vi "SampleGetIDMultiple.vi"() -> ()   [LabVIEW 2016]
panel:
  out "Device number":i32
  out "Identification List":string[](array[string])
  out "DeviceKey List Out":string[](array[string])
  out "error out":errorcluster
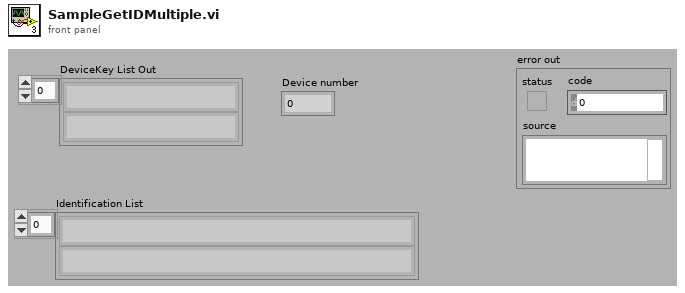
[diagram p1: front panel]
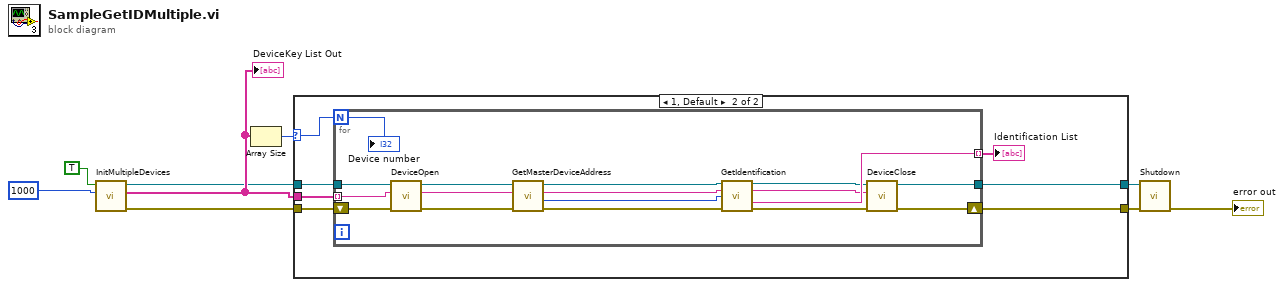
[diagram p0: block diagram]
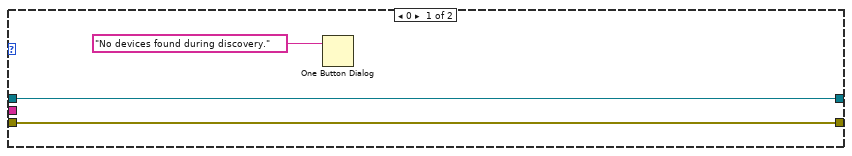
[diagram p2: hidden frame]
diagram:
  n1 = call "InitMultipleDevices.vi"("msecDelayForDiscovery"=1000, "logging"=TRUE) -> ("error out"=w1:errorcluster, "DeviceKey List Out"=w5:string[], "CmdLib Out"=w2:refnum<k24>)  [unwired: 3 in]
  "DeviceKey List Out" <- w5
  n2 = Array Size(array=w5) -> (size(s)=w6:i32)
  n3 = case shown="1, Default" w6 {
    selector: w6 -> [_ w19]
    tunnel: w5 -> [_ w18]
    tunnel: w2 -> [w11 w17]
    tunnel: w1 -> [w12 w16]
    tunnel: [w12 w15] -> w4
    tunnel: [w11 w14] -> w3
    frame 0 {
      n4 = One Button Dialog(message="No devices found during discovery.") -> ()  [unwired: 1 in, 1 out]
    }
    frame 1, Default {
      n5 = for {
        N: w19 -> [w20]
        tunnel: w18 -> [w32] mode=indexing
        tunnel: [w36] -> w13 mode=indexing
        tunnel: w17 -> [w35]
        tunnel: [w34] -> w14
        shift-right: [w30] -> w15
        shift-left: w16 -> [w31]
        n6 = call "DeviceOpen.vi"("error in (no error)"=w31, "DeviceKey In"=w32, "CmdLib In"=w35) -> ("error out"=w25:errorcluster, "DeviceKey Out"=w26:string, "CmdLib Out"=w27:refnum<k24>)  [unwired: 2 in]
        n7 = call "GetMasterDeviceAddress.vi"("error in (no error)"=w25, "DeviceKey In"=w26, "CmdLib In"=w27) -> ("error out"=w21:errorcluster, "Device Address"=w24:i32, "DeviceKey Out"=w23:string, "CmdLib Out"=w22:refnum<k24>)  [unwired: 1 in]
        n8 = call "GetIdentification.vi"("CmdLib In"=w22, "DeviceKey In"=w23, "Device Address In"=w24, "error in (no error)"=w21) -> ("CmdLib Out"=w33:refnum<k24>, "DeviceKey Out"=w28:string, "Identification"=w36:string, "error out"=w29:errorcluster)  [unwired: 7 in, 1 out]
        n9 = call "DeviceClose.vi"("error in (no error)"=w29, "DeviceKey In"=w28, "CmdLib In"=w33) -> ("error out"=w30:errorcluster, "CmdLib Out"=w34:refnum<k24>)  [unwired: 2 in, 1 out]
        "Device number" <- w20
      }
      "Identification List" <- w13
    }
  }
  n10 = call "Shutdown.vi"("error in (no error)"=w4, "CmdLib In"=w3) -> ("error out"=→"error out":errorcluster)  [unwired: 4 in, 1 out]
